vi "Write TagY.vi"(2 "error in (no error)":errorcluster, 3 "TagY":dbl, 4 "Tag in":refnum<class "Tag.lvclass">) -> (0 "error out":errorcluster, 1 "Tag out":refnum<class "Tag.lvclass">)   [LabVIEW 2014, in "Tag.lvclass"]
uses:
  Tag.lvclass
  Tag.lvclass/Tag.ctl
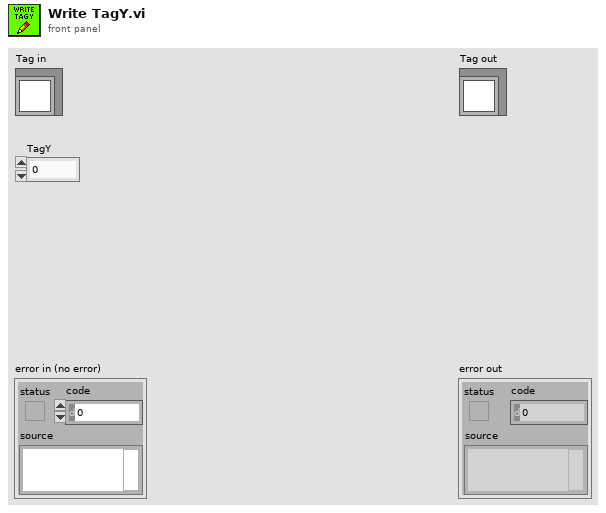
[diagram p1: front panel]
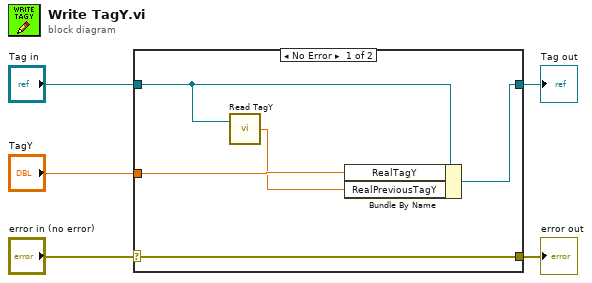
[diagram p0: block diagram]
diagram:
  n1 = case shown="No Error" "error in (no error)" {
    selector: "error in (no error)" -> [w10 w11]
    tunnel: [w10 w11] -> w4
    tunnel: [w9 w12] -> w2
    tunnel: "Tag in" -> [w7 w12]
    tunnel: "TagY" -> [w8 _]
    frame No Error {
      n2 = call-dynamic "Read TagY.vi"("Tag in"=w7) -> ("RealTagY"=w6:dbl)  [unwired: 1 in, 2 out]
      n3 = Bundle By Name(cluster=w7, "RealTagY"=w8, "RealPreviousTagY"=w6) -> (w9:refnum<class "Tag.lvclass">)
    }
    frame Error {
    }
  }
  "error out" <- w4
  "Tag out" <- w2
